vi "Array of Double_ASCII String To Data.vi"(8 "error in (no error)":errorcluster, 9 "Default":cluster{"DBL Array":dbl[]}, 11 "Value":string) -> (0 "error out":errorcluster, 3 "Data":cluster{"DBL Array":dbl[]})   [LabVIEW 2020, in "Current Value Table(Rebuild).lvlib"]
doc: "This VI converts data stored on disk as an ascii string into the correct data type. This VI must perform the opposite operation to the DataToASCIIString function."
uses:
  Current Value Table(Rebuild).lvlib
  Errors/Generate Error.vi
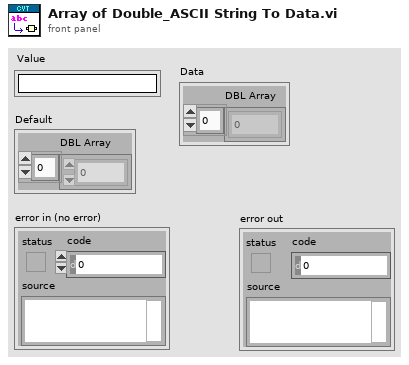
[diagram p1: front panel]
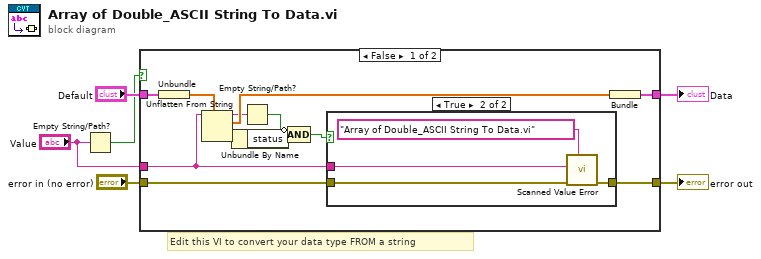
[diagram p0: block diagram]
diagram:
  # "Edit this VI to convert your data type FROM a string"
  n1 = Empty String/Path?(string/path="Value") -> (empty?=w3:bool)
  n2 = case shown="False" w3 {
    tunnel: "Default" -> [w17 w25]
    tunnel: "Value" -> [w15 _]
    tunnel: [w13 w25] -> w1
    tunnel: "error in (no error)" -> [w8 w24]
    tunnel: [w18 w24] -> w5
    frame False {
      n3 = Unbundle(w17) -> ("DBL Array"=w16:dbl[])
      n4 = Unflatten From String(type=w16, binary string=w15) -> (rest of the binary string=w9:string, value=w14:dbl[], error out=w10:errorcluster)  [unwired: 3 in]
      n5 = Unbundle By Name(w10) -> ("status"=w7:bool)
      n6 = Empty String/Path?(string/path=w9) -> (empty?=w11:bool)
      n7 = Compound Arithmetic op=AND(invert w11, w7) -> (w12:bool)
      n8 = case shown="True" w12 {
        tunnel: [w19 w23] -> w18
        tunnel: w15 -> [_ w22]
        tunnel: w8 -> [w19 w21]
        frame False {
        }
        frame True {
          n9 = call "Scanned Value Error.vi"("caller name"="Array of Double_ASCII String To Data.vi", "error in (no error)"=w21, "Value"=w22) -> ("error out"=w23:errorcluster)  [unwired: 8 in]
        }
      }
      n10 = Bundle("DBL Array"=w14) -> (w13:cluster{"DBL Array":dbl[]})  [unwired: 1 in]
    }
    frame True {
    }
  }
  "error out" <- w5
  "Data" <- w1
